vi "path_septag.vi"() -> ()   [LabVIEW 2021]
panel:
  in  "Path":path=path "file"
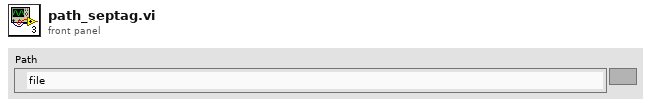
[diagram p1: front panel]
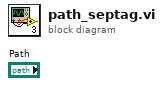
[diagram p0: block diagram]
diagram:
